vi "TIFF_Format_JSON.vi"(8 "error in (no error)":errorcluster, 11 "Description":string) -> (0 "error out":errorcluster, 3 "Channel_Cluster_Array OUT":T1(array[cluster]))   [LabVIEW 2025]
uses:
  <vilib>/addons/_JKI.lib/Serialization/JSON/JKI JSON Serialization.lvlib
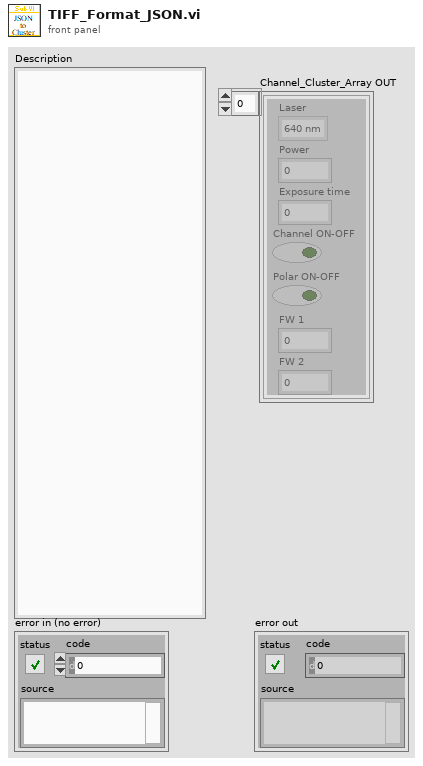
[diagram p1: front panel]
types:
  T1 = cluster{"Laser":enum16{"640 nm", "561 nm"}, "Power":u8, "Exposure time":dbl, "Channel ON-OFF":bool, "Polar ON-OFF":bool, "FW 1":u16, "FW 2":u16}[]
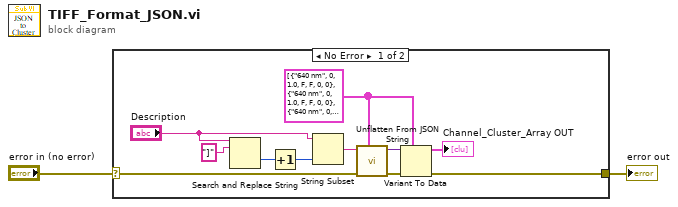
[diagram p0: block diagram]
diagram:
  n1 = case shown="No Error" "error in (no error)" {
    selector: "error in (no error)" -> [w4 w14]
    tunnel: [w7 w14] -> w2
    frame No Error {
      w8 = T1 [{"Laser"=enum."640 nm", "Power"=0, "Exposure time"=1.0, "Channel ON-OFF"=FALSE, "Polar ON-OFF"=FALSE, "FW 1"=0, "FW 2"=0}, {"Laser"=enum."640 nm", "Power"=0, "Exposure time"=1.0, "Channel ON-OFF"=FALSE, "Polar ON-OFF"=FALSE, "FW 1"=0, "FW 2"=0}, {"Laser"=enum."640 nm", "Power"=0, "Exposure time"=1.0, "Channel ON-OFF"=FALSE, "Polar ON-OFF"=FALSE, "FW 1"=0, "FW 2"=0}] ("Channel_Cluster_Array OUT")
      n2 = Search and Replace String(input string="Description", search string="]") -> (offset past replacement=w11:i32)  [unwired: 6 in, 3 out]
      n3 = Increment(x=w11) -> (x+1=w12:i32)
      n4 = String Subset(string="Description", length (rest)=w12) -> (substring=w13:string)  [unwired: 1 in]
      n5 = call <vilib>:"Unflatten From JSON String.vi"("Type and Defaults"=w8, "error in"=w4, "JSON String"=w13) -> ("error out"=w5:errorcluster, "Variant"=w6:variant)  [unwired: 7 in]
      n6 = Variant To Data(error in=w5, type=w8, Variant=w6) -> (data=→"Channel_Cluster_Array OUT":T1, error out=w7:errorcluster)
    }
    frame Error {
    }
  }
  "error out" <- w2
